vi "Init.vi"(8 "error in (no error)":errorcluster, 11 "Data in":refnum<class "Fault-Injection Bus.lvclass">) -> (0 "error out":errorcluster, 3 "Data out":refnum<class "Fault-Injection Bus.lvclass">)   [LabVIEW 2021, in "Fault-Injection Bus.lvclass"]
doc: "Abstract Data Classes 2.1.1.12\nTim Streeter - TSA\nCopyright (c) 2024, TSA"
uses:
  Fault-Injection Bus.lvclass
  C:/Users/Tim/Documents/GitHub/Omni-Bus/Source/Omni-Bus/Bus Access/Bus_Access.lvclass
  Fault-Injection Bus.lvclass/Fault-Injection Bus.ctl
  Omni-Bus/Bus Access/Bus_Access.lvclass/Bus_Access.ctl
  <vilib>/TSA/Abstract Data Classes/Abs_Types/Value/Abs_Value.lvclass
  C:/Program Files (x86)/National Instruments/LabVIEW 2021/vi.lib/TSA/Abstract Data Classes/Abs_Types/Type/Abs_Type.lvclass
  Support/Value Type/Boolean/Fault-Injection_Boolean.lvclass
  C:/Program Files (x86)/National Instruments/LabVIEW 2021/vi.lib/TSA/Abstract Data Classes/Abs_Types/Value/Abs_Value.lvclass
  Support/Value Type/DBL/Fault-Injection_DBL.lvclass
  Support/Value Type/SGL/Fault-Injection_SGL.lvclass
  Support/Value Type/EXT/Fault-Injection_EXT.lvclass
  Support/Value Type/CSGL/Fault-Injection_CSGL.lvclass
  Support/Value Type/CDBL/Fault-Injection_CDBL.lvclass
  Support/Value Type/CEXT/Fault-Injection_CEXT.lvclass
  Support/Value Type/U8/Fault-Injection_U8.lvclass
  Support/Value Type/U16/Fault-Injection_U16.lvclass
  Support/Value Type/U32/Fault-Injection_U32.lvclass
  Support/Value Type/U64/Fault-Injection_U64.lvclass
  Support/Value Type/I8/Fault-Injection_I8.lvclass
  Support/Value Type/I16/Fault-Injection_I16.lvclass
  Support/Value Type/I32/Fault-Injection_I32.lvclass
  Support/Value Type/I64/Fault-Injection_I64.lvclass
  Support/Value Type/Variant/Fault-Injection_Variant.lvclass
  Support/Value Type/STR/Fault-Injection_STR.lvclass
  Support/Value Type/WFM/Fault-Injection_WFM.lvclass
  Support/Value Type/Time/Fault-Injection_Time.lvclass
  Omni-Bus/Bus Access/Properties/Read Values.vi
  Omni-Bus/Bus Access/Properties/Read Tag Root.vi
  Omni-Bus/Bus Access/Properties/Read Tags.vi
  Properties/Read Buses.vi
  Properties/Write Data DVR.vi
  Properties/Write Arm.vi
  Properties/Write Buses.vi
  Omni-Bus/Bus Access/Properties/Write Values.vi
  Omni-Bus/Bus Access/Properties/Write Tag Root.vi
  Omni-Bus/Bus Access/Properties/Write Tags.vi
  Omni-Bus/Bus Access/Bus_Access.lvclass
  <vilib>/TSA/Abstract Data Classes/Abs_Types/Type/Abs_Type.lvclass
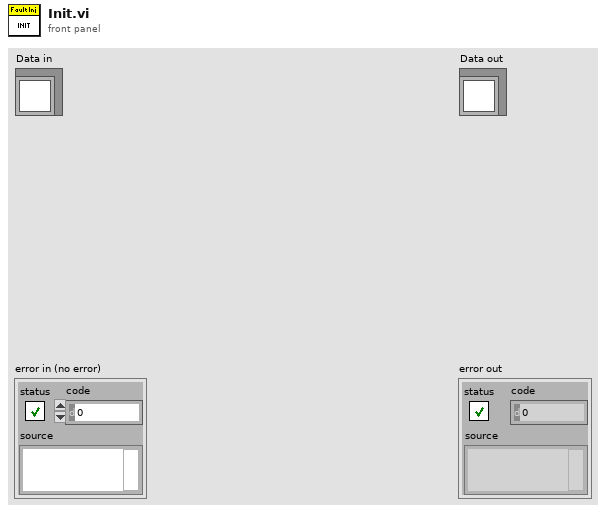
[diagram p1: front panel]
types:
  T1 = typedef "Fault-Injection Bus.lvclass/DVR Type.ctl" = cluster{"Boolean":refnum<data-value>, "String":refnum<data-value>, "DBL":refnum<data-value>, "SGL":refnum<data-value>, "EXT":refnum<data-value>, "U8":refnum<data-value>, "U16":refnum<data-value>, "U32":refnum<data-value>, "U64":refnum<data-value>, "I8":refnum<data-value>, "I16":refnum<data-value>, "I32":refnum<data-value>, "I64":refnum<data-value>, "CDBL":refnum<data-value>, "CSGL":refnum<data-value>, "CEXT":refnum<data-value>, "Time":refnum<data-value>, "Variant":refnum<data-value>, "Waveform":refnum<data-value>, "Type":refnum<data-value>}
  T2 = typedef "NI_Data Type.lvlib/Data Type.ctl" = enum8{"Invalid Type", "Void", "I8", "I16", "I32", "I64", "U8", "U16", "U32", "U64", "Single Float", "Double Float", "Extended Float", "Single Complex", "Double Complex", "Extended Complex", "Enum U8", "Enum U16", "Enum U32", "Enum U64", "Single Float With Unit", "Double Float With Unit", "Extended Float With Unit", "Single Complex with Unit", "Double Complex with Unit", "Extended Complex with Unit", "Boolean", "String", "Path", "Picture", "Tag", "Array", "Cluster", "Variant", "LV Variant", "Waveform", "Timestamp", "Digital Waveform", "Digital Data", "ExpressData", "Refnum", "External Data", "VI", "Poly VI", "LabVIEW Class Instance", "Fixed Point", "Set Collection", "Map Collection"}
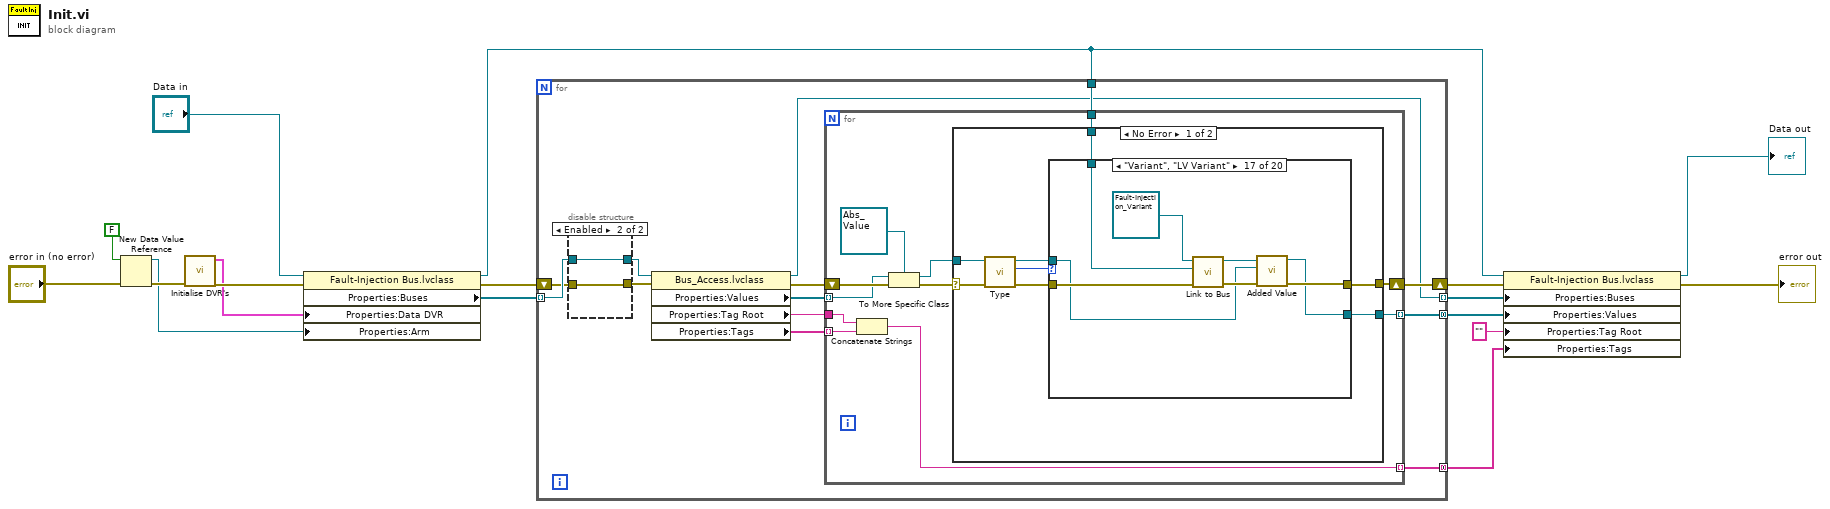
[diagram p0: block diagram]
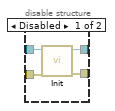
[diagram p2: hidden frame]
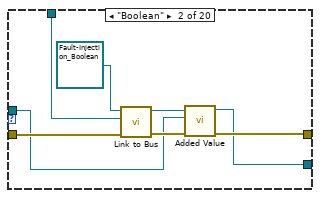
[diagram p4: hidden frame]
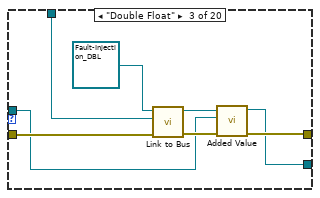
[diagram p5: hidden frame]
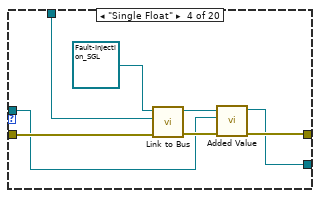
[diagram p6: hidden frame]
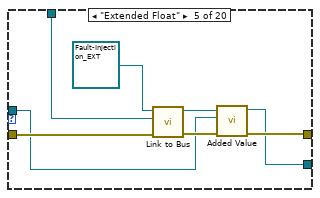
[diagram p7: hidden frame]
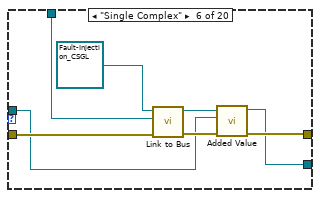
[diagram p8: hidden frame]
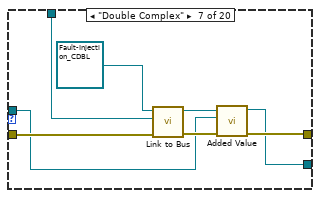
[diagram p9: hidden frame]
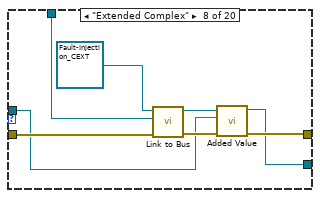
[diagram p10: hidden frame]
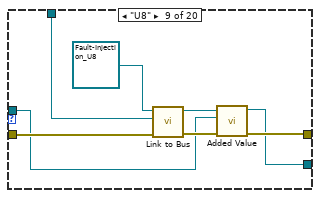
[diagram p11: hidden frame]
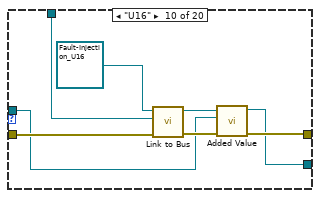
[diagram p12: hidden frame]
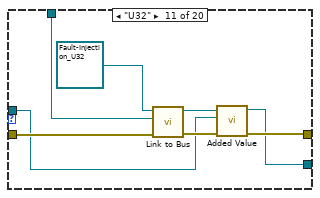
[diagram p13: hidden frame]
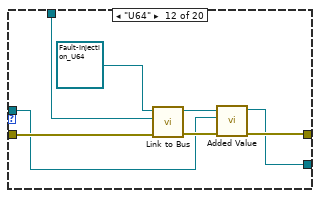
[diagram p14: hidden frame]
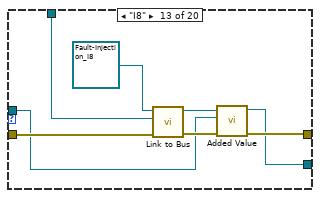
[diagram p15: hidden frame]
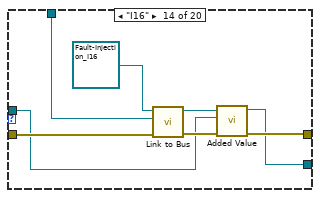
[diagram p16: hidden frame]
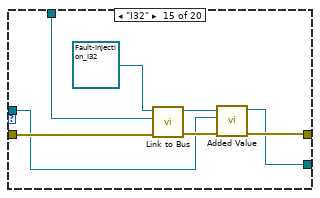
[diagram p17: hidden frame]
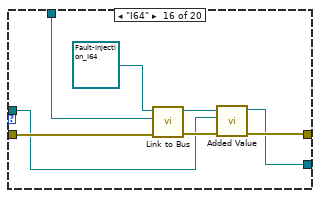
[diagram p18: hidden frame]
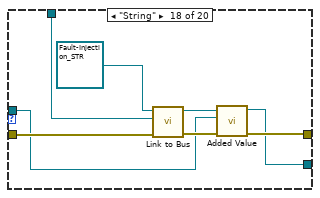
[diagram p19: hidden frame]
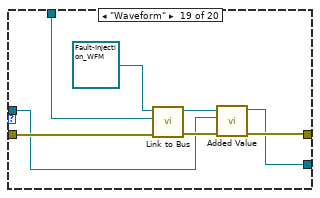
[diagram p20: hidden frame]
diagram:
  n1 = New Data Value Reference(data value=FALSE, error in="error in (no error)") -> (data value reference=w2:refnum<data-value>, error out=w5:errorcluster)
  n2 = call "Initialise DVR's.vi"("error in (no error)"=w5) -> ("error out"=w7:errorcluster, "Type"=w6:T1)  [unwired: 9 in]
  n3 = property class="Fault-Injection Bus.lvclass"(reference="Data in", error in=w7, "Properties:Data DVR"=w6, "Properties:Arm"=w2) -> (reference out=w8:refnum<class "Fault-Injection Bus.lvclass">, error out=w15:errorcluster, "Properties:Buses"=w16:refnum<class "Bus_Access.lvclass">[])
  n4 = for {
    tunnel: w16 -> [w22] mode=indexing
    shift-right: [w25] -> w14
    shift-left: w15 -> [w21]
    tunnel: [w26] -> w13 mode=concatenating
    tunnel: [w24] -> w11 mode=concatenating
    tunnel: w8 -> [w23]
    tunnel: [w18] -> w1 mode=indexing
    n5 = disable-structure shown="Enabled" {
      disable-tunnel: w22 -> [w34 w35]
      disable-tunnel: w21 -> [w33 w36]
      disable-tunnel: [w32 w36] -> w20
      disable-tunnel: [w31 w35] -> w19
      frame Disabled {
        n6 = call-dynamic "Init.vi"("error in (no error)"=w33, "Data in"=w34) -> ("error out"=w32:errorcluster, "Data out"=w31:refnum<class "Bus_Access.lvclass">)  [unwired: 8 in]
      }
      frame Enabled {
      }
    }
    n7 = property class="Bus_Access.lvclass"(reference=w19, error in=w20) -> (reference out=w18:refnum<class "Bus_Access.lvclass">, error out=w29:errorcluster, "Properties:Values"=w30:refnum<class "Abs_Type.lvclass">[], "Properties:Tag Root"=w28:string, "Properties:Tags"=w27:string[])
    n8 = for {
      tunnel: w30 -> [w46] mode=indexing
      shift-right: [w42] -> w25
      shift-left: w29 -> [w47]
      tunnel: w28 -> [w40]
      tunnel: w27 -> [w41] mode=indexing
      tunnel: [w37] -> w26 mode=indexing
      tunnel: [w39] -> w24 mode=indexing
      tunnel: w23 -> [w38]
      n9 = Concatenate Strings(w40, w41) -> (w37:string)
      n10 = To More Specific Class(target class=refnum<class "Abs_Value.lvclass"> refnum ("Type in"), reference=w46, error in=w47) -> (specific class reference=w43:refnum<class "Abs_Value.lvclass">, error out=w44:errorcluster)
      n11 = case shown="No Error" w44 {
        selector: w44 -> [w55 w212]
        tunnel: w43 -> [w54 w210]
        tunnel: [w49 w211] -> w42
        tunnel: [w50 w210] -> w39
        tunnel: w38 -> [w48 _]
        frame No Error {
          n12 = call-dynamic "Type.vi"("error in (no error)"=w55, "Element in"=w54) -> ("error out"=w51:errorcluster, "Type"=w53:T2, "Element out"=w52:refnum<class "Abs_Value.lvclass">)  [unwired: 7 in]
          n13 = case shown="\"Variant\", \"LV Variant\"" w53 {
            tunnel: w52 -> [w57 w60 w69 w77 w85 w93 w101 w109 w117 w125 w133 w141 w149 w157 w165 w173 w181 w189 w197 w205]
            tunnel: w51 -> [w56 w65 w73 w81 w89 w97 w105 w113 w121 w129 w137 w145 w153 w161 w169 w177 w185 w193 w201 w209]
            tunnel: [w57 w58 w67 w75 w83 w91 w99 w107 w115 w123 w131 w139 w147 w155 w163 w171 w179 w187 w195 w203] -> w50
            tunnel: [w56 w59 w68 w76 w84 w92 w100 w108 w116 w124 w132 w140 w148 w156 w164 w172 w180 w188 w196 w204] -> w49
            tunnel: w48 -> [_ w63 w72 w80 w88 w96 w104 w112 w120 w128 w136 w144 w152 w160 w168 w176 w184 w192 w200 w208]
            frame "Invalid Type", Default {
              # "Even if the type isn't supported\nit needs to be included so it doesn't\nbreak the code"
            }
            frame "Boolean" {
              n14 = call-dynamic "Link to Bus.vi"("error in (no error)"=w65, "Fault-Injection Bus.lvclass"=w63, "Local Bus_DBL in"=refnum<class "Fault-Injection_Boolean.lvclass"> refnum ("Fault-Injection_Boolean.lvclass")) -> ("error out"=w61:errorcluster, "Local Bus_DBL out"=w62:refnum<class "Fault-Injection_Boolean.lvclass">)  [unwired: 7 in]
              n15 = call-dynamic "Added Value.vi"("error in (no error)"=w61, "Element in"=w60, "Fault-Injection_Boolean in"=w62) -> ("error out"=w59:errorcluster, "Fault-Injection_Boolean out"=w58:refnum<class "Fault-Injection_Boolean.lvclass">)  [unwired: 7 in]
            }
            frame "Double Float" {
              n16 = call-dynamic "Link to Bus.vi"("error in (no error)"=w73, "Fault-Injection Bus.lvclass"=w72, "Local Bus_DBL in"=refnum<class "Fault-Injection_DBL.lvclass"> refnum ("Fault-Injection_DBL.lvclass")) -> ("error out"=w70:errorcluster, "Local Bus_DBL out"=w71:refnum<class "Fault-Injection_DBL.lvclass">)  [unwired: 7 in]
              n17 = call-dynamic "Added Value.vi"("error in (no error)"=w70, "Element in"=w69, "Fault-Injection_Boolean in"=w71) -> ("error out"=w68:errorcluster, "Fault-Injection_Boolean out"=w67:refnum<class "Fault-Injection_DBL.lvclass">)  [unwired: 7 in]
            }
            frame "Single Float" {
              n18 = call-dynamic "Link to Bus.vi"("error in (no error)"=w81, "Fault-Injection Bus.lvclass"=w80, "Local Bus_DBL in"=refnum<class "Fault-Injection_SGL.lvclass"> refnum ("Fault-Injection_SGL.lvclass")) -> ("error out"=w78:errorcluster, "Local Bus_DBL out"=w79:refnum<class "Fault-Injection_SGL.lvclass">)  [unwired: 7 in]
              n19 = call-dynamic "Added Value.vi"("error in (no error)"=w78, "Element in"=w77, "Fault-Injection_Boolean in"=w79) -> ("error out"=w76:errorcluster, "Fault-Injection_Boolean out"=w75:refnum<class "Fault-Injection_SGL.lvclass">)  [unwired: 7 in]
            }
            frame "Extended Float" {
              n20 = call-dynamic "Link to Bus.vi"("error in (no error)"=w89, "Fault-Injection Bus.lvclass"=w88, "Local Bus_DBL in"=refnum<class "Fault-Injection_EXT.lvclass"> refnum ("Fault-Injection_EXT.lvclass")) -> ("error out"=w86:errorcluster, "Local Bus_DBL out"=w87:refnum<class "Fault-Injection_EXT.lvclass">)  [unwired: 7 in]
              n21 = call-dynamic "Added Value.vi"("error in (no error)"=w86, "Element in"=w85, "Fault-Injection_Boolean in"=w87) -> ("error out"=w84:errorcluster, "Fault-Injection_Boolean out"=w83:refnum<class "Fault-Injection_EXT.lvclass">)  [unwired: 7 in]
            }
            frame "Single Complex" {
              n22 = call-dynamic "Link to Bus.vi"("error in (no error)"=w97, "Fault-Injection Bus.lvclass"=w96, "Local Bus_DBL in"=refnum<class "Fault-Injection_CSGL.lvclass"> refnum ("Fault-Injection_CSGL.lvclass")) -> ("error out"=w94:errorcluster, "Local Bus_DBL out"=w95:refnum<class "Fault-Injection_CSGL.lvclass">)  [unwired: 7 in]
              n23 = call-dynamic "Added Value.vi"("error in (no error)"=w94, "Element in"=w93, "Fault-Injection_Boolean in"=w95) -> ("error out"=w92:errorcluster, "Fault-Injection_Boolean out"=w91:refnum<class "Fault-Injection_CSGL.lvclass">)  [unwired: 7 in]
            }
            frame "Double Complex" {
              n24 = call-dynamic "Link to Bus.vi"("error in (no error)"=w105, "Fault-Injection Bus.lvclass"=w104, "Local Bus_DBL in"=refnum<class "Fault-Injection_CDBL.lvclass"> refnum ("Fault-Injection_CDBL.lvclass")) -> ("error out"=w102:errorcluster, "Local Bus_DBL out"=w103:refnum<class "Fault-Injection_CDBL.lvclass">)  [unwired: 7 in]
              n25 = call-dynamic "Added Value.vi"("error in (no error)"=w102, "Element in"=w101, "Fault-Injection_Boolean in"=w103) -> ("error out"=w100:errorcluster, "Fault-Injection_Boolean out"=w99:refnum<class "Fault-Injection_CDBL.lvclass">)  [unwired: 7 in]
            }
            frame "Extended Complex" {
              n26 = call-dynamic "Link to Bus.vi"("error in (no error)"=w113, "Fault-Injection Bus.lvclass"=w112, "Local Bus_DBL in"=refnum<class "Fault-Injection_CEXT.lvclass"> refnum ("Fault-Injection_CEXT.lvclass")) -> ("error out"=w110:errorcluster, "Local Bus_DBL out"=w111:refnum<class "Fault-Injection_CEXT.lvclass">)  [unwired: 7 in]
              n27 = call-dynamic "Added Value.vi"("error in (no error)"=w110, "Element in"=w109, "Fault-Injection_Boolean in"=w111) -> ("error out"=w108:errorcluster, "Fault-Injection_Boolean out"=w107:refnum<class "Fault-Injection_CEXT.lvclass">)  [unwired: 7 in]
            }
            frame "U8" {
              n28 = call-dynamic "Link to Bus.vi"("error in (no error)"=w121, "Fault-Injection Bus.lvclass"=w120, "Local Bus_DBL in"=refnum<class "Fault-Injection_U8.lvclass"> refnum ("Fault-Injection_U8.lvclass")) -> ("error out"=w118:errorcluster, "Local Bus_DBL out"=w119:refnum<class "Fault-Injection_U8.lvclass">)  [unwired: 7 in]
              n29 = call-dynamic "Added Value.vi"("error in (no error)"=w118, "Element in"=w117, "Fault-Injection_Boolean in"=w119) -> ("error out"=w116:errorcluster, "Fault-Injection_Boolean out"=w115:refnum<class "Fault-Injection_U8.lvclass">)  [unwired: 7 in]
            }
            frame "U16" {
              n30 = call-dynamic "Link to Bus.vi"("error in (no error)"=w129, "Fault-Injection Bus.lvclass"=w128, "Local Bus_DBL in"=refnum<class "Fault-Injection_U16.lvclass"> refnum ("Fault-Injection_U16.lvclass")) -> ("error out"=w126:errorcluster, "Local Bus_DBL out"=w127:refnum<class "Fault-Injection_U16.lvclass">)  [unwired: 7 in]
              n31 = call-dynamic "Added Value.vi"("error in (no error)"=w126, "Element in"=w125, "Fault-Injection_Boolean in"=w127) -> ("error out"=w124:errorcluster, "Fault-Injection_Boolean out"=w123:refnum<class "Fault-Injection_U16.lvclass">)  [unwired: 7 in]
            }
            frame "U32" {
              n32 = call-dynamic "Link to Bus.vi"("error in (no error)"=w137, "Fault-Injection Bus.lvclass"=w136, "Local Bus_DBL in"=refnum<class "Fault-Injection_U32.lvclass"> refnum ("Fault-Injection_U32.lvclass")) -> ("error out"=w134:errorcluster, "Local Bus_DBL out"=w135:refnum<class "Fault-Injection_U32.lvclass">)  [unwired: 7 in]
              n33 = call-dynamic "Added Value.vi"("error in (no error)"=w134, "Element in"=w133, "Fault-Injection_Boolean in"=w135) -> ("error out"=w132:errorcluster, "Fault-Injection_Boolean out"=w131:refnum<class "Fault-Injection_U32.lvclass">)  [unwired: 7 in]
            }
            frame "U64" {
              n34 = call-dynamic "Link to Bus.vi"("error in (no error)"=w145, "Fault-Injection Bus.lvclass"=w144, "Local Bus_DBL in"=refnum<class "Fault-Injection_U64.lvclass"> refnum ("Fault-Injection_U64.lvclass")) -> ("error out"=w142:errorcluster, "Local Bus_DBL out"=w143:refnum<class "Fault-Injection_U64.lvclass">)  [unwired: 7 in]
              n35 = call-dynamic "Added Value.vi"("error in (no error)"=w142, "Element in"=w141, "Fault-Injection_Boolean in"=w143) -> ("error out"=w140:errorcluster, "Fault-Injection_Boolean out"=w139:refnum<class "Fault-Injection_U64.lvclass">)  [unwired: 7 in]
            }
            frame "I8" {
              n36 = call-dynamic "Link to Bus.vi"("error in (no error)"=w153, "Fault-Injection Bus.lvclass"=w152, "Local Bus_DBL in"=refnum<class "Fault-Injection_I8.lvclass"> refnum ("Fault-Injection_I8.lvclass")) -> ("error out"=w150:errorcluster, "Local Bus_DBL out"=w151:refnum<class "Fault-Injection_I8.lvclass">)  [unwired: 7 in]
              n37 = call-dynamic "Added Value.vi"("error in (no error)"=w150, "Element in"=w149, "Fault-Injection_Boolean in"=w151) -> ("error out"=w148:errorcluster, "Fault-Injection_Boolean out"=w147:refnum<class "Fault-Injection_I8.lvclass">)  [unwired: 7 in]
            }
            frame "I16" {
              n38 = call-dynamic "Link to Bus.vi"("error in (no error)"=w161, "Fault-Injection Bus.lvclass"=w160, "Local Bus_DBL in"=refnum<class "Fault-Injection_I16.lvclass"> refnum ("Fault-Injection_I16.lvclass")) -> ("error out"=w158:errorcluster, "Local Bus_DBL out"=w159:refnum<class "Fault-Injection_I16.lvclass">)  [unwired: 7 in]
              n39 = call-dynamic "Added Value.vi"("error in (no error)"=w158, "Element in"=w157, "Fault-Injection_Boolean in"=w159) -> ("error out"=w156:errorcluster, "Fault-Injection_Boolean out"=w155:refnum<class "Fault-Injection_I16.lvclass">)  [unwired: 7 in]
            }
            frame "I32" {
              n40 = call-dynamic "Link to Bus.vi"("error in (no error)"=w169, "Fault-Injection Bus.lvclass"=w168, "Local Bus_DBL in"=refnum<class "Fault-Injection_I32.lvclass"> refnum ("Fault-Injection_I32.lvclass")) -> ("error out"=w166:errorcluster, "Local Bus_DBL out"=w167:refnum<class "Fault-Injection_I32.lvclass">)  [unwired: 7 in]
              n41 = call-dynamic "Added Value.vi"("error in (no error)"=w166, "Element in"=w165, "Fault-Injection_Boolean in"=w167) -> ("error out"=w164:errorcluster, "Fault-Injection_Boolean out"=w163:refnum<class "Fault-Injection_I32.lvclass">)  [unwired: 7 in]
            }
            frame "I64" {
              n42 = call-dynamic "Link to Bus.vi"("error in (no error)"=w177, "Fault-Injection Bus.lvclass"=w176, "Local Bus_DBL in"=refnum<class "Fault-Injection_I64.lvclass"> refnum ("Fault-Injection_I64.lvclass")) -> ("error out"=w174:errorcluster, "Local Bus_DBL out"=w175:refnum<class "Fault-Injection_I64.lvclass">)  [unwired: 7 in]
              n43 = call-dynamic "Added Value.vi"("error in (no error)"=w174, "Element in"=w173, "Fault-Injection_Boolean in"=w175) -> ("error out"=w172:errorcluster, "Fault-Injection_Boolean out"=w171:refnum<class "Fault-Injection_I64.lvclass">)  [unwired: 7 in]
            }
            frame "Variant", "LV Variant" {
              n44 = call-dynamic "Link to Bus.vi"("error in (no error)"=w185, "Fault-Injection Bus.lvclass"=w184, "Local Bus_DBL in"=refnum<class "Fault-Injection_Variant.lvclass"> refnum ("Fault-Injection_Variant.lvclass")) -> ("error out"=w182:errorcluster, "Local Bus_DBL out"=w183:refnum<class "Fault-Injection_Variant.lvclass">)  [unwired: 7 in]
              n45 = call-dynamic "Added Value.vi"("error in (no error)"=w182, "Element in"=w181, "Fault-Injection_Boolean in"=w183) -> ("error out"=w180:errorcluster, "Fault-Injection_Boolean out"=w179:refnum<class "Fault-Injection_Variant.lvclass">)  [unwired: 7 in]
            }
            frame "String" {
              n46 = call-dynamic "Link to Bus.vi"("error in (no error)"=w193, "Fault-Injection Bus.lvclass"=w192, "Local Bus_DBL in"=refnum<class "Fault-Injection_STR.lvclass"> refnum ("Fault-Injection_STR.lvclass")) -> ("error out"=w190:errorcluster, "Local Bus_DBL out"=w191:refnum<class "Fault-Injection_STR.lvclass">)  [unwired: 7 in]
              n47 = call-dynamic "Added Value.vi"("error in (no error)"=w190, "Element in"=w189, "Fault-Injection_Boolean in"=w191) -> ("error out"=w188:errorcluster, "Fault-Injection_Boolean out"=w187:refnum<class "Fault-Injection_STR.lvclass">)  [unwired: 7 in]
            }
            frame "Waveform" {
              n48 = call-dynamic "Link to Bus.vi"("error in (no error)"=w201, "Fault-Injection Bus.lvclass"=w200, "Local Bus_DBL in"=refnum<class "Fault-Injection_WFM.lvclass"> refnum ("Fault-Injection_WFM.lvclass")) -> ("error out"=w198:errorcluster, "Local Bus_DBL out"=w199:refnum<class "Fault-Injection_WFM.lvclass">)  [unwired: 7 in]
              n49 = call-dynamic "Added Value.vi"("error in (no error)"=w198, "Element in"=w197, "Fault-Injection_Boolean in"=w199) -> ("error out"=w196:errorcluster, "Fault-Injection_Boolean out"=w195:refnum<class "Fault-Injection_WFM.lvclass">)  [unwired: 7 in]
            }
            frame "Timestamp" {
              n50 = call-dynamic "Link to Bus.vi"("error in (no error)"=w209, "Fault-Injection Bus.lvclass"=w208, "Local Bus_DBL in"=refnum<class "Fault-Injection_Time.lvclass"> refnum ("Fault-Injection_Time.lvclass")) -> ("error out"=w206:errorcluster, "Local Bus_DBL out"=w207:refnum<class "Fault-Injection_Time.lvclass">)  [unwired: 7 in]
              n51 = call-dynamic "Added Value.vi"("error in (no error)"=w206, "Element in"=w205, "Fault-Injection_Boolean in"=w207) -> ("error out"=w204:errorcluster, "Fault-Injection_Boolean out"=w203:refnum<class "Fault-Injection_Time.lvclass">)  [unwired: 7 in]
            }
          }
        }
        frame Error {
          # "Not a value type\nso we can't inject\na fault"
          n52 = call <vilib>:"Clear Errors.vi"("error in (no error)"=w212) -> ("error out"=w211:errorcluster)  [unwired: 5 in, 1 out]
        }
      }
    }
  }
  n53 = property class="Fault-Injection Bus.lvclass"(reference=w8, error in=w14, "Properties:Buses"=w1, "Properties:Values"=w11, "Properties:Tag Root"="" ("Tag Root"), "Properties:Tags"=w13) -> (reference out=→"Data out":refnum<class "Fault-Injection Bus.lvclass">, error out=→"error out":errorcluster)
